vi "PH_uOPA_DelayController.Set Default.vi"(0 "i ref in":refnum<vi>, 5 "error in":errorcluster) -> (14 "i ref out":refnum<vi>, 19 "error out":errorcluster)   [LabVIEW 2014, in "PH_uOPA_DelayController.lvlib"]
doc: "This VI sets the hardware to default configuration."
uses:
  PH_uOPA_DelayController.lvlib
  PH_Devices/PH_TKTDS-30xx/PH_TKTDS-30xx.Trigger Config.ctl
  PH_Devices/PH_TKTDS-30xx/PH_TKTDS-30xx.Acquisition Config.ctl
  PH_Devices/PH_TKTDS-30xx/PH_TKTDS-30xx.Channel Config.ctl
  PH_Devices/PH_TKTDS-30xx/PH_TKTDS-30xx.Waveform Limits.ctl
  PH_Devices/PH_TKTDS-30xx/PH_TKTDS-30xx.lvlib
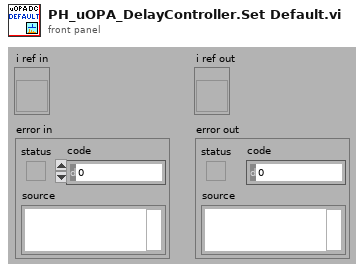
[diagram p1: front panel]
types:
  T1 = typedef "PH_TKTDS-30xx.lvlib/PH_TKTDS-30xx.Acquisition Config.ctl" = cluster{"Time base":dbl, "Record Length":u16, "Start Time":dbl, "Type":i32, "Continuous":bool}
  T2 = typedef "PH_TKTDS-30xx.lvlib/PH_TKTDS-30xx.Trigger Config.ctl" = cluster{"Source":string, "Slope":i32, "Level [V]":dbl}
  T3 = typedef "PH_TKTDS-30xx.lvlib/PH_TKTDS-30xx.i attribute.ctl" = cluster{"Default VISA Resource":string, "VISA Resource Name":refnum<visa-resource-name>, "Revision":cluster{"Instrument Driver":string, "Instrument Firmware":string}, "Selftest":cluster{"Result":u32, "Message":string}, "Channels":T4[], "Trigger Configuration":T2, "Acquisition Configuration":T1, "Fetched Waveforms":T6[], "GUI Refs":T7, "State":T8, "Error Message":string, "Allow Prdc Loop?":bool}
  T4 = typedef "PH_TKTDS-30xx.lvlib/PH_TKTDS-30xx.Channel Config.ctl" = cluster{"Channel Name":string, "Input Impedance":string, "Max Input Frequency":string, "Vertical Coupling":i32, "Channel Enabled":bool, "Probe Attenuation":dbl, "Vertical Range":dbl, "Vertical Offset":dbl, "Waveform Limits":T5}
  T5 = typedef "PH_TKTDS-30xx.lvlib/PH_TKTDS-30xx.Waveform Limits.ctl" = cluster{"Start":i32, "End":i32}
  T6 = typedef "PH_TKTDS-30xx.lvlib/PH_TKTDS-30xx.fetched Waveform.ctl" = cluster{"Source":string, "Actual Points":u32, "Initial X":dbl, "X Increment":dbl, "Waveform Array":dbl[]}
  T7 = typedef "PH_TKTDS-30xx.lvlib/PH_TKTDS-30xx.GUI Refs.ctl" = cluster{"Trigger":refnum<vi>, "Acquisition":refnum<vi>, "State":refnum<vi>, "Delete":refnum<vi>, "Channel to be positioned":refnum<vi>, "Postion":refnum<vi>, "Display Intensity":refnum<vi>, "VISA Resource":refnum<vi>, "Channels":refnum<vi>[], "Graphs":refnum<vi>[]}
  T8 = typedef "PH_StatusHandler.lvlib/PH_StatusHandler.Status.ctl" = i16
  T9 = cluster{"GUI Element Name":string, "Chan Settings":T4}
  T10 = cluster{"GUI Element Name":string, "Chan Settings":T4}[]
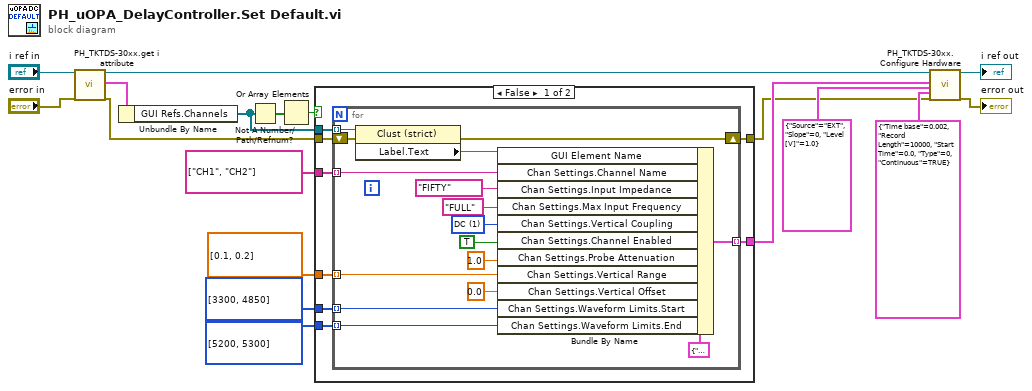
[diagram p0: block diagram]
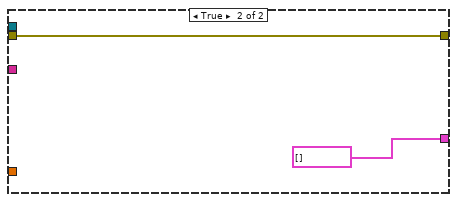
[diagram p2: hidden frame]
diagram:
  w7 = dbl[] [0.1, 0.2] items=["1mV"=0.001, "2mV"=0.002, "5mV"=0.005, "10mV"=0.01, "20mV"=0.02, "50mV"=0.05, "100mV"=0.1, "200mV"=0.2, "500mV"=0.5, "1V"=1.0]
  n1 = call "PH_TKTDS-30xx.get i attribute.vi"("i ref in"="i ref in", "error in (no error)"="error in") -> ("i ref out"=w12:refnum<vi>, "i attribute"=w11:T3, "error out"=w9:errorcluster)  [unwired: 15 in]
  n2 = Unbundle By Name(w11) -> ("GUI Refs.Channels"=w5:refnum<vi>[])
  n3 = Not A Number/Path/Refnum?(number/path/refnum=w5) -> (NaN/Path/Refnum?=w4:bool[])
  n4 = Or Array Elements(Boolean array=w4) -> (logical OR=w3:bool)
  n5 = case shown="False" w3 {
    tunnel: [w26 T10 []] -> w10
    tunnel: w9 -> [w25 w43]
    tunnel: [w24 w43] -> w8
    tunnel: w7 -> [w23 _]
    tunnel: string[] ["CH1", "CH2"] -> [w22 _]
    tunnel: w5 -> [w21 _]
    tunnel: i32[] [3300, 4850] -> [w20 _]
    tunnel: i32[] [5200, 5300] -> [w19 _]
    frame False {
      n6 = for {
        tunnel: w21 -> [w42] mode=indexing
        shift-right: [w40] -> w24
        shift-left: w25 -> [w41]
        tunnel: [w39] -> w26 mode=indexing
        tunnel: w23 -> [w38] mode=indexing
        tunnel: w22 -> [w37] mode=indexing
        tunnel: w20 -> [w28] mode=indexing
        tunnel: w19 -> [w27] mode=indexing
        w30 = 1 items=["AC", "DC", "GND"] ("Vertical Coupling")
        n7 = property class="Clust (strict)"(reference=w42, error in=w41) -> (error out=w40:errorcluster, "Label.Text"=w36:string)  [unwired: 1 out]
        n8 = Bundle By Name(cluster=T9 {"GUI Element Name"="", "Chan Settings"={"Channel Name"="CH1", "Input Impedance"="MEG", "Max Input Frequency"="TWENTY", "Vertical Coupling"=1, "Channel Enabled"=TRUE, "Probe Attenuation"=1.0, "Vertical Range"=100.0, "Vertical Offset"=0.0, "Waveform Limits"={"Start"=1, "End"=10000}}} ("Channel Settings"), "GUI Element Name"=w36, "Chan Settings.Channel Name"=w37, "Chan Settings.Input Impedance"="FIFTY" ("Input Impedance"), "Chan Settings.Max Input Frequency"="FULL" ("Max Input Frequency"), "Chan Settings.Vertical Coupling"=w30, "Chan Settings.Channel Enabled"=TRUE, "Chan Settings.Probe Attenuation"=1.0, "Chan Settings.Vertical Range"=w38, "Chan Settings.Vertical Offset"=0.0, "Chan Settings.Waveform Limits.Start"=w28, "Chan Settings.Waveform Limits.End"=w27) -> (w39:T9)
      }
    }
    frame True {
    }
  }
  n9 = call "PH_TKTDS-30xx.Configure Hardware.vi"("i ref in"=w12, "Channels Sets"=w10, "Trigger Settings"=T2 {"Source"="EXT", "Slope"=0, "Level [V]"=1.0}, "Acqu Settings"=T1 {"Time base"=0.002, "Record Length"=10000, "Start Time"=0.0, "Type"=0, "Continuous"=TRUE}, "error in"=w8) -> ("i ref out"=→"i ref out":refnum<vi>, "error out"=→"error out":errorcluster)  [unwired: 13 in]
